vi "Get Context.vi"(8 "error in (no error)":errorcluster, 11 "Process In":refnum<class "Debug Process.lvclass">) -> (0 "error out":errorcluster, 1 "Top Level?":bool, 2 "Context":refnum<class "Debug Process.lvclass">, 3 "Process Out":refnum<class "Debug Process.lvclass">)   [LabVIEW 2020, in "Debug Process.lvclass"]
doc: "Returns the context of the process. If the process is top level application an error is returned."
uses:
  Debug Process.lvclass
  Debug Process.lvclass/Debug Process.ctl
  <vilib>/Utility/error.llb/Clear Errors.vi
  <vilib>/Utility/error.llb/Error Cluster From Error Code.vi
  <vilib>/ErrorRing/Error Ring.xnode
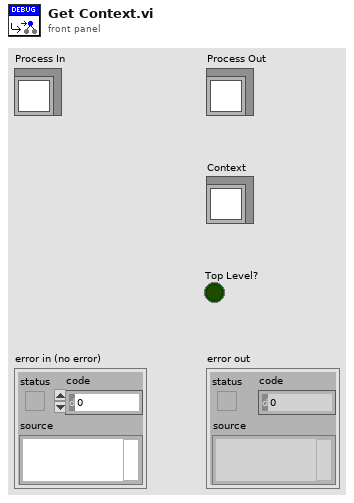
[diagram p1: front panel]
types:
  T1 = typedef "Debug Process.lvclass/Lifecycle State.ctl" = enum16{"Uninitialized", "Initialized", "Started", "Running", "Stopped", "Finished"}
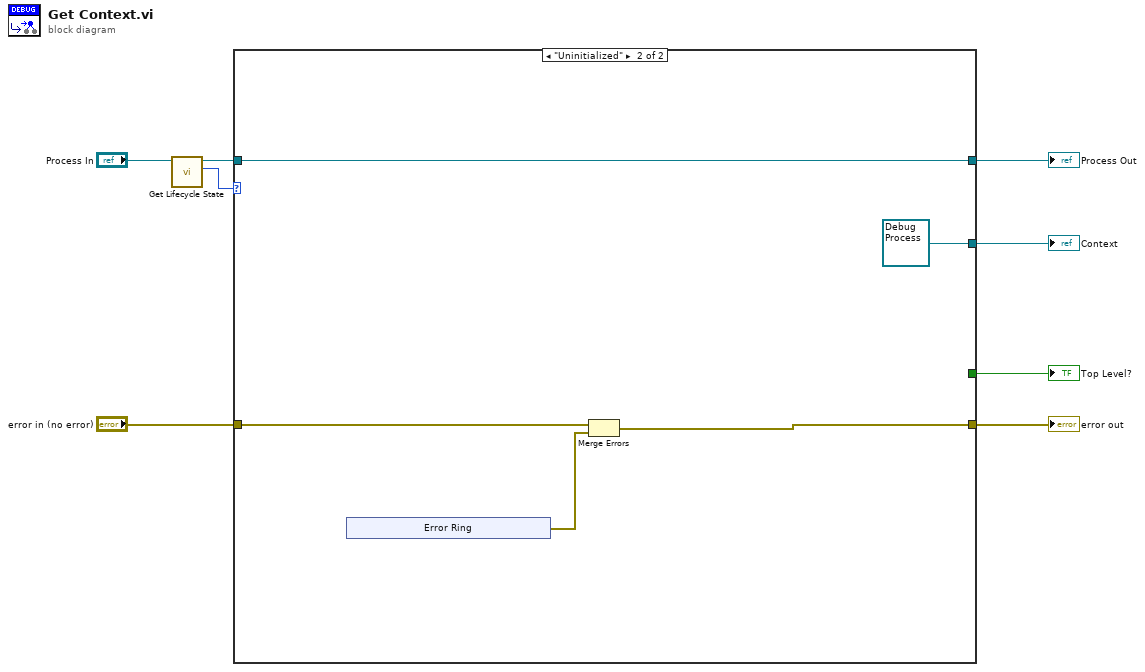
[diagram p0: block diagram]
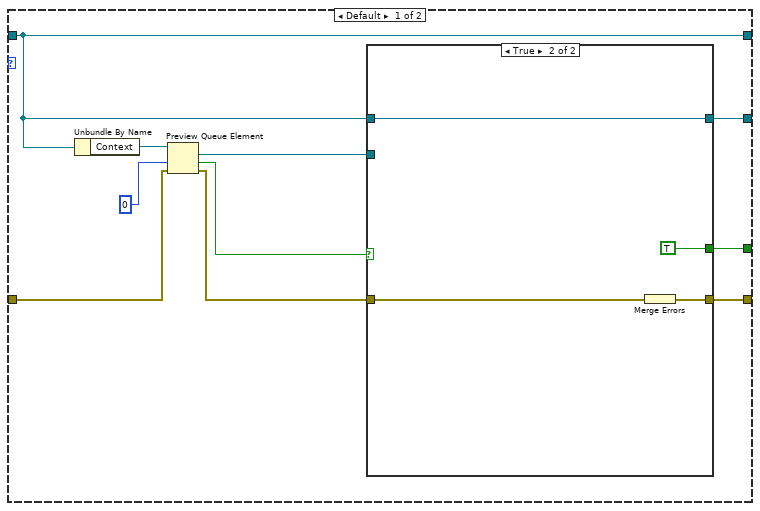
[diagram p2: hidden frame]
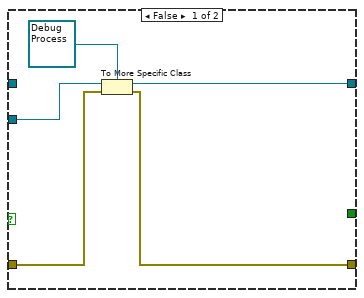
[diagram p3: hidden frame]
diagram:
  n1 = call "Get Lifecycle State.vi"("Process In"="Process In") -> ("Lifecycle State"=w2:T1, "Process Out"=w3:refnum<class "Debug Process.lvclass">)  [unwired: 7 in, 2 out]
  n2 = case shown="\"Uninitialized\"" w2 {
    tunnel: w3 -> [w10 w30]
    tunnel: [w10 w30] -> w7
    tunnel: [w18 refnum<class "Debug Process.lvclass"> refnum ("Error Handler")] -> w6
    tunnel: [w17 w29] -> w5
    tunnel: "error in (no error)" -> [w12 w32]
    tunnel: [w9 _] -> w4
    frame Default {
      n3 = Unbundle By Name(w10) -> ("Context"=w16:refnum<queue>)
      n4 = Preview Queue Element(queue=w16, timeout in ms (-1)=0, error in (no error)=w12) -> (element=w13:refnum<class>, timed out?=w11:bool, error out=w15:errorcluster)  [unwired: 1 out]
      n5 = case shown="True" w11 {
        tunnel: [w23 w25] -> w18
        tunnel: [w19 w26] -> w17
        tunnel: w13 -> [w21 _]
        tunnel: w15 -> [w20 w27]
        tunnel: w10 -> [_ w25]
        tunnel: [_ TRUE] -> w9
        frame False {
          n6 = To More Specific Class(target class=refnum<class "Debug Process.lvclass"> refnum ("Error Handler"), reference=w21, error in=w20) -> (specific class reference=w23:refnum<class "Debug Process.lvclass">, error out=w19:errorcluster)
        }
        frame True {
          n7 = Merge Errors(w27) -> (w26:errorcluster)
        }
      }
    }
    frame "Uninitialized" {
      n8 = xnode "Error Ring"() -> ("error out"=w28:errorcluster)
      n9 = Merge Errors(w32, w28) -> (w29:errorcluster)
    }
  }
  "error out" <- w5
  "Process Out" <- w7
  "Context" <- w6
  "Top Level?" <- w4
